vi "Read Aout Cfactor.vi"(8 "error in (no error)":errorcluster, 11 "VISA resource name":refnum<visa-resource-name>) -> (0 "error out":errorcluster, 2 "aout cfactor":cluster{"CFactorC":dbl, "CFactorL":dbl}, 3 "VISA resource name out":refnum<visa-resource-name>)   [LabVIEW 2025, in "Andeen-Hagerling 2700A.lvlib"]
doc: "Return the input to output voltage conversion factor for the\ncapacitance and loss voltage output channels in V/pF and\nV/jpF respectively."
uses:
  Andeen-Hagerling 2700A.lvlib
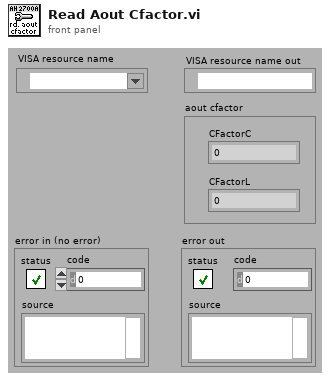
[diagram p1: front panel]
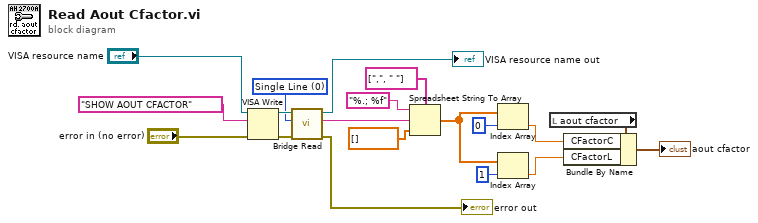
[diagram p0: block diagram]
diagram:
  w1 = u16 0 items=["Single Line", "Multi-Line"] ("Multiline")
  n1 = VISA Write(VISA resource name="VISA resource name", write buffer="SHOW AOUT CFACTOR" ("command"), error in (no error)="error in (no error)") -> (VISA resource name out=w12:refnum<visa-resource-name>, error out=w11:errorcluster)  [unwired: 1 out]
  n2 = call "Bridge Read.vi"("error in (no error)"=w11, "multiline"=w1, "VISA resource name"=w12) -> ("error out"=→"error out":errorcluster, "read buffer"=w10:string, "VISA resource name out"=→"VISA resource name out":refnum<visa-resource-name>)  [unwired: 6 in]
  n3 = Spreadsheet String To Array(delimiter (Tab)=string[] [",", " "], format string="%.; %f", spreadsheet string=w10, array type (2D Dbl)=dbl[] []) -> (array=w5:dbl[])
  n4 = Index Array(array=w5, index=0) -> (element=w3:dbl)
  n5 = Index Array(array=w5, index=1) -> (element=w4:dbl)
  n6 = local read "aout cfactor"() -> (w9:cluster{"CFactorC":dbl, "CFactorL":dbl})
  n7 = Bundle By Name(cluster=w9, "CFactorC"=w3, "CFactorL"=w4) -> (→"aout cfactor":cluster{"CFactorC":dbl, "CFactorL":dbl})
